vi "SalvarDadosTemporario.vi"(7 "FileName":string, 8 "ErrorIn":errorcluster, 9 "Path":path, 10 "Read/Write(Read)":enum16{"Read", "Write"}(ring), 11 "DataInp":variant) -> (0 "ErrorOut":errorcluster, 3 "DataOut":variant)   [LabVIEW 2019]
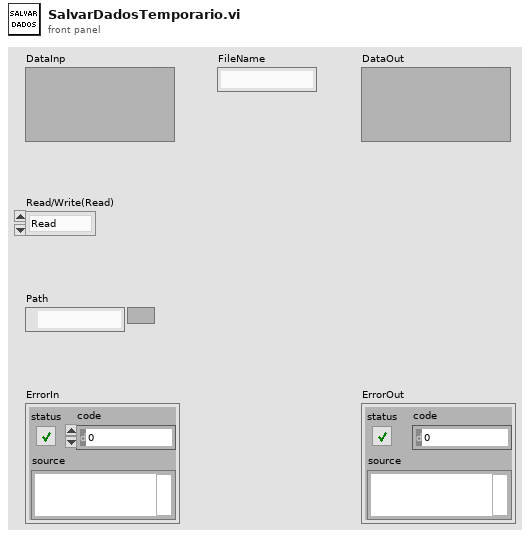
[diagram p1: front panel]
types:
  T1 = enum16{"open", "replace", "create", "open or create", "replace or create", "replace or create with confirmation"}
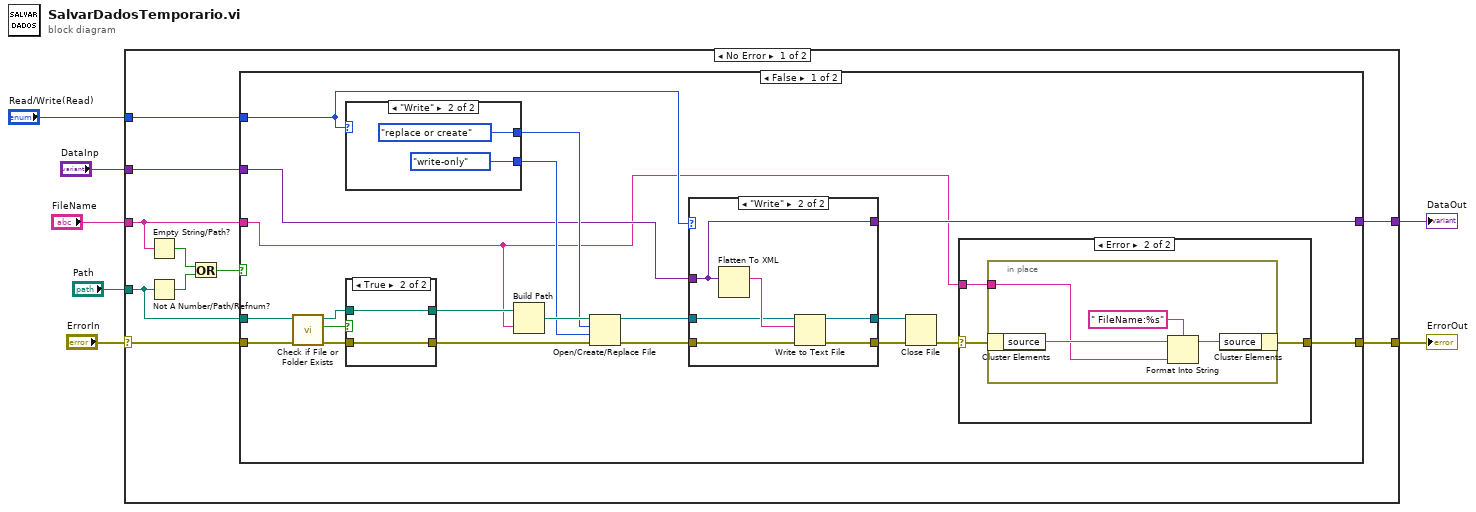
[diagram p0: block diagram]
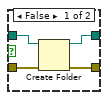
[diagram p3: hidden frame]
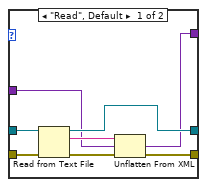
[diagram p4: hidden frame]
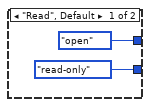
[diagram p5: hidden frame]
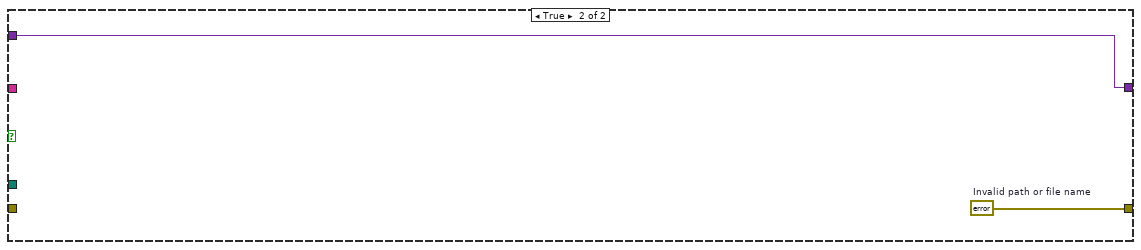
[diagram p6: hidden frame]
diagram:
  n1 = case shown="No Error" "ErrorIn" {
    selector: "ErrorIn" -> [w14 w73]
    tunnel: [w13 w73] -> w6
    tunnel: "Read/Write(Read)" -> [w17 _]
    tunnel: "DataInp" -> [w16 w72]
    tunnel: [w15 w72] -> w3
    tunnel: "FileName" -> [w12 _]
    tunnel: "Path" -> [w8 _]
    frame No Error {
      n2 = Empty String/Path?(string/path=w12) -> (empty?=w10:bool)
      n3 = Not A Number/Path/Refnum?(number/path/refnum=w8) -> (NaN/Path/Refnum?=w9:bool)
      n4 = Or(x=w10, y=w9) -> (x .or. y?=w11:bool)
      n5 = case shown="False" w11 {
        tunnel: w17 -> [w30 _]
        tunnel: w16 -> [w29 w71]
        tunnel: [w28 w71] -> w15
        tunnel: w14 -> [w20 _]
        tunnel: w12 -> [w22 _]
        tunnel: [w21 w70] -> w13
        tunnel: w8 -> [w19 _]
        frame False {
          n6 = call <vilib>:"Check if File or Folder Exists.vi"("error in (no error)"=w20, "path"=w19) -> ("error out"=w27:errorcluster, "file or folder exists?"=w25:bool, "dup path"=w26:path)  [unwired: 7 in]
          n7 = case shown="\"Write\"" w30 {
            tunnel: [T1."open" ("operation (0:open)") T1."replace or create" ("operation (0:open)")] -> w36
            tunnel: [enum16{"read/write", "read-only", "write-only"}."read-only" ("access (0:read/write)") enum16{"read/write", "read-only", "write-only"}."write-only" ("access (0:read/write)")] -> w34
            frame "Read", Default {
            }
            frame "Write" {
            }
          }
          n8 = case shown="True" w25 {
            tunnel: w26 -> [w49 w51]
            tunnel: w27 -> [w48 w50]
            tunnel: [w47 w51] -> w24
            tunnel: [w46 w50] -> w23
            frame False {
              n9 = Create Folder(path (use dialog)=w49, error in=w48) -> (created path=w47:path, error out=w46:errorcluster)  [unwired: 1 in, 1 out]
            }
            frame True {
            }
          }
          n10 = Build Path(base path=w24, name or relative path=w22) -> (appended path=w37:path)
          n11 = Open/Create/Replace File(file path (use dialog)=w37, error in=w23, operation (0:open)=w36, access (0:read/write)=w34) -> (refnum out=w33:refnum<file>, error out=w35:errorcluster)  [unwired: 2 in, 1 out]
          n12 = case shown="\"Write\"" w30 {
            tunnel: w35 -> [w59 w65]
            tunnel: w33 -> [w58 w60]
            tunnel: [w57 w62] -> w32
            tunnel: w29 -> [w55 w63]
            tunnel: [w54 w63] -> w28
            tunnel: [w52 w61] -> w31
            frame "Read", Default {
              n13 = Read from Text File(file (use dialog)=w58, error in=w59) -> (refnum out=w57:refnum<file>, text=w56:string, error out=w53:errorcluster)  [unwired: 2 in, 1 out]
              n14 = Unflatten From XML(xml string=w56, type=w55, error in (no error)=w53) -> (value=w54:variant, error out=w52:errorcluster)
            }
            frame "Write" {
              n15 = Flatten To XML(anything=w63) -> (xml string=w64:string)
              n16 = Write to Text File(file (use dialog)=w60, text=w64, error in=w65) -> (refnum out=w62:refnum<file>, error out=w61:errorcluster)  [unwired: 1 in, 1 out]
            }
          }
          n17 = Close File(refnum=w32, error in=w31) -> (error out=w18:errorcluster)  [unwired: 1 out]
          n18 = case shown="Error" w18 {
            selector: w18 -> [w38 w39]
            tunnel: w22 -> [_ w41]
            tunnel: [w38 w40] -> w21
            frame No Error {
            }
            frame Error {
              n19 = in-place {
                in-place-border: w41 -> [w42]
                n20 = in-place-cluster #1(w39) -> ("source"=w44:string)
                n21 = Format Into String(format string=" FileName:%s", initial string=w44, w42) -> (resulting string=w43:string)  [unwired: 1 in, 1 out]
                n22 = in-place-cluster #1("source"=w43) -> (w40:errorcluster)
              }
            }
          }
        }
        frame True {
          w70 = errorcluster {"status"=TRUE, "code"=999, "source"="Invalid path or file name"}  # Invalid path or file name
        }
      }
    }
    frame Error {
    }
  }
  "ErrorOut" <- w6
  "DataOut" <- w3
